vi "校准对话框.vi"(8 "error in (no error)":errorcluster, 11 "VISA Refnum in":refnum<visa-resource-name>) -> (0 "error out":errorcluster, 3 "VISA resource name out":refnum<visa-resource-name>)   [LabVIEW 2015, in "keysight.lvclass"]
uses:
  keysight.lvclass
  E5071C/Agilent ENA Series/Agilent ENA Series.lvlib
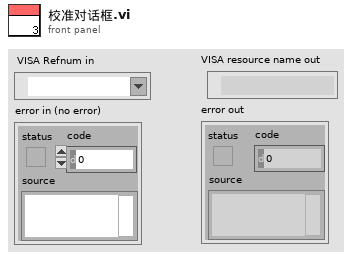
[diagram p1: front panel]
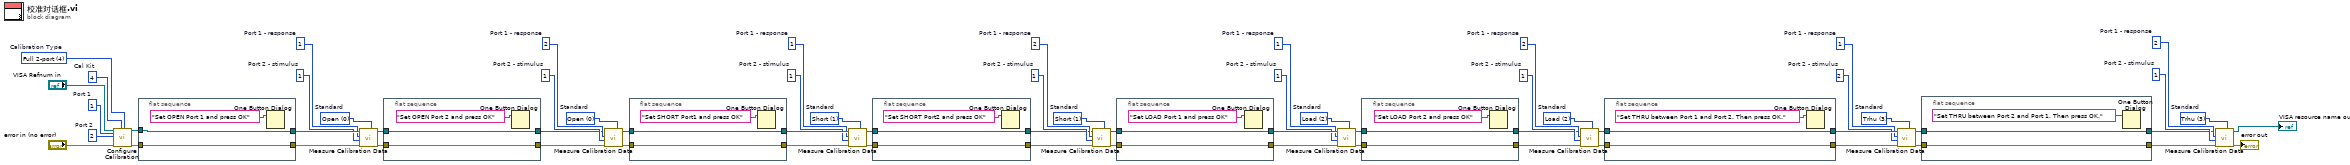
[diagram p0: block diagram]
diagram:
  w10 = u16 3 items=["Open", "Short", "Load", "Trhu", "Isolation"]  # Standard
  w12 = 1  # Port 2 - stimulus
  w11 = 2  # Port 1 - response
  w19 = u16 3 items=["Open", "Short", "Load", "Trhu", "Isolation"]  # Standard
  w15 = 2  # Port 2 - stimulus
  w16 = 1  # Port 1 - response
  w22 = u16 2 items=["Open", "Short", "Load", "Trhu", "Isolation"]  # Standard
  w26 = 1  # Port 2 - stimulus
  w25 = 2  # Port 1 - response
  w33 = u16 2 items=["Open", "Short", "Load", "Trhu", "Isolation"]  # Standard
  w29 = 1  # Port 2 - stimulus
  w30 = 1  # Port 1 - response
  w36 = u16 1 items=["Open", "Short", "Load", "Trhu", "Isolation"]  # Standard
  w40 = 1  # Port 2 - stimulus
  w39 = 2  # Port 1 - response
  w47 = u16 1 items=["Open", "Short", "Load", "Trhu", "Isolation"]  # Standard
  w43 = 1  # Port 2 - stimulus
  w44 = 1  # Port 1 - response
  w48 = u16 0 items=["Open", "Short", "Load", "Trhu", "Isolation"]  # Standard
  w49 = u16 0 items=["Open", "Short", "Load", "Trhu", "Isolation"]  # Standard
  w55 = 1  # Port 2 - stimulus
  w54 = 2  # Port 1 - response
  w56 = 1  # Port 2 - stimulus
  w57 = 1  # Port 1 - response
  w61 = 2  # Port 2
  w62 = 1  # Port 1
  w63 = u16 4 items=["Open", "Short", "Through", "1-port", "Full 2-port", "Full 3-port", "Full 4-port"]  # Calibration Type
  w64 = 4  # Cal Kit
  n1 = call "Configure Calibration.vi"("VISA resource name"="VISA Refnum in", "Port 1 (1)"=w62, "Port 2 (1)"=w61, "error in (no error)"="error in (no error)", "Cal Kit (1)"=w64, "Calibration Type (6: Full 4-port)"=w63) -> ("VISA resource name out"=w5:refnum<visa-resource-name>, "error out"=w4:errorcluster)  [unwired: 12 in]
  n2 = flat-sequence {
    tunnel: w5 -> [w66]
    tunnel: w4 -> [w65]
    tunnel: [w65] -> w58
    tunnel: [w66] -> w59
    frame #0 {
      n3 = One Button Dialog(message="Set OPEN Port 1 and press OK") -> ()  [unwired: 1 in, 1 out]
    }
  }
  n4 = call "Measure Calibration Data.vi"("Standard (0: Open)"=w49, "error in (no error)"=w58, "Port 2 - stimulus (2)"=w56, "Port 1 - response (1)"=w57, "VISA resource name"=w59) -> ("error out"=w50:errorcluster, "VISA resource name out"=w51:refnum<visa-resource-name>)  [unwired: 5 in]
  n5 = flat-sequence {
    tunnel: w51 -> [w69]
    tunnel: w50 -> [w68]
    tunnel: [w68] -> w53
    tunnel: [w69] -> w52
    frame #0 {
      n6 = One Button Dialog(message="Set OPEN Port 2 and press OK") -> ()  [unwired: 1 in, 1 out]
    }
  }
  n7 = call "Measure Calibration Data.vi"("Standard (0: Open)"=w48, "error in (no error)"=w53, "Port 2 - stimulus (2)"=w55, "Port 1 - response (1)"=w54, "VISA resource name"=w52) -> ("error out"=w41:errorcluster, "VISA resource name out"=w42:refnum<visa-resource-name>)  [unwired: 5 in]
  n8 = flat-sequence {
    tunnel: w42 -> [w72]
    tunnel: w41 -> [w71]
    tunnel: [w71] -> w45
    tunnel: [w72] -> w46
    frame #0 {
      n9 = One Button Dialog(message="Set SHORT Port1 and press OK") -> ()  [unwired: 1 in, 1 out]
    }
  }
  n10 = call "Measure Calibration Data.vi"("Standard (0: Open)"=w47, "error in (no error)"=w45, "Port 2 - stimulus (2)"=w43, "Port 1 - response (1)"=w44, "VISA resource name"=w46) -> ("error out"=w34:errorcluster, "VISA resource name out"=w35:refnum<visa-resource-name>)  [unwired: 5 in]
  n11 = flat-sequence {
    tunnel: w35 -> [w75]
    tunnel: w34 -> [w74]
    tunnel: [w74] -> w38
    tunnel: [w75] -> w37
    frame #0 {
      n12 = One Button Dialog(message="Set SHORT Port2 and press OK") -> ()  [unwired: 1 in, 1 out]
    }
  }
  n13 = call "Measure Calibration Data.vi"("Standard (0: Open)"=w36, "error in (no error)"=w38, "Port 2 - stimulus (2)"=w40, "Port 1 - response (1)"=w39, "VISA resource name"=w37) -> ("error out"=w27:errorcluster, "VISA resource name out"=w28:refnum<visa-resource-name>)  [unwired: 5 in]
  n14 = flat-sequence {
    tunnel: w28 -> [w78]
    tunnel: w27 -> [w77]
    tunnel: [w77] -> w31
    tunnel: [w78] -> w32
    frame #0 {
      n15 = One Button Dialog(message="Set LOAD Port 1 and press OK") -> ()  [unwired: 1 in, 1 out]
    }
  }
  n16 = call "Measure Calibration Data.vi"("Standard (0: Open)"=w33, "error in (no error)"=w31, "Port 2 - stimulus (2)"=w29, "Port 1 - response (1)"=w30, "VISA resource name"=w32) -> ("error out"=w20:errorcluster, "VISA resource name out"=w21:refnum<visa-resource-name>)  [unwired: 5 in]
  n17 = flat-sequence {
    tunnel: w21 -> [w81]
    tunnel: w20 -> [w80]
    tunnel: [w80] -> w24
    tunnel: [w81] -> w23
    frame #0 {
      n18 = One Button Dialog(message="Set LOAD Port 2 and press OK") -> ()  [unwired: 1 in, 1 out]
    }
  }
  n19 = call "Measure Calibration Data.vi"("Standard (0: Open)"=w22, "error in (no error)"=w24, "Port 2 - stimulus (2)"=w26, "Port 1 - response (1)"=w25, "VISA resource name"=w23) -> ("error out"=w13:errorcluster, "VISA resource name out"=w14:refnum<visa-resource-name>)  [unwired: 5 in]
  n20 = flat-sequence {
    tunnel: w14 -> [w84]
    tunnel: w13 -> [w83]
    tunnel: [w83] -> w17
    tunnel: [w84] -> w18
    frame #0 {
      n21 = One Button Dialog(message="Set THRU between Port 1 and Port 2. Then press OK.") -> ()  [unwired: 1 in, 1 out]
    }
  }
  n22 = call "Measure Calibration Data.vi"("Standard (0: Open)"=w19, "error in (no error)"=w17, "Port 2 - stimulus (2)"=w15, "Port 1 - response (1)"=w16, "VISA resource name"=w18) -> ("error out"=w8:errorcluster, "VISA resource name out"=w9:refnum<visa-resource-name>)  [unwired: 5 in]
  n23 = flat-sequence {
    tunnel: w9 -> [w87]
    tunnel: w8 -> [w86]
    tunnel: [w86] -> w6
    tunnel: [w87] -> w7
    frame #0 {
      n24 = One Button Dialog(message="Set THRU between Port 2 and Port 1. Then press OK.") -> ()  [unwired: 1 in, 1 out]
    }
  }
  n25 = call "Measure Calibration Data.vi"("Standard (0: Open)"=w10, "error in (no error)"=w6, "Port 2 - stimulus (2)"=w12, "Port 1 - response (1)"=w11, "VISA resource name"=w7) -> ("error out"=→"error out":errorcluster, "VISA resource name out"=→"VISA resource name out":refnum<visa-resource-name>)  [unwired: 5 in]
